vi "Project.vi"() -> ()   [LabVIEW 2015]
uses:
  <vilib>/express/express analysis/Spectral/Block/exnSpectralBlock spectral measurements RMS poly.vi
  <vilib>/express/express analysis/Spectral/Block/exnSpectralBlock spectral measurements RMS WFM.vi
  <vilib>/Analysis/BLAS.llb/dasum - Absolute Values Sum (DBL).vi
  <vilib>/express/express analysis/Spectral/XNode/ExpressSpectralMeasurementsBlockNode.xnode
  <vilib>/Analysis/NI_AALBLAS.lvlib
panel:
  out "Fourier Spectrum":cluster{"f0":dbl, "df":dbl, "magnitude":dbl[]}(graph)={"f0"=0.0, "df"=1.0, "magnitude"=[0.042500606468979685, 0.5367467757567798, 0.3916687019986553, 0.298960203892999, 0.6710643612299553, 6.999534465420016, 1.1013196943424124, 0.18951549536081805, 0.4623568704519078, 0.15713994611889348, 0.20038906279151222, 0.12934410129286392, 0.2068645394551969, 0.23302748208959884, 0.22176371644713225, 0.08751545175582917, 0.13513069757467858, 0.06308830540493562, 0.39375621048035264, 0.01345553332772048, 7.1986582467475, 0.1538936478758767, 0.11526828636783537, 0.06727117464447396, 0.2733833694778588, 0.08171771490184758, 0.12959665685604613, 0.08906888825527193, 0.2742960376602098, 0.10825189397057566, 0.09709745409455775, 0.2003023769713194, 0.24422273703495245, 0.154193230936854, 0.02225848069093769, 0.029518364210050947, 0.2694030850949449, 0.2545730206460508, 0.03493546942572119, 0.09895571125122078, 0.2284739144767194, 0.15064812633383587, 0.1284930441857229, 0.14474851518272724, 0.17923036833316625, 0.19036481120281232, 0.17636492792839045, 0.12006498175113303, 0.17954194318688638, 0.2106284617581408, 0.28299962121792593, 0.23538566157052568, 0.24018555003640282, 0.21640041472758512, 0.15124757101737055, 0.41949661945335315, 0.26981879550897725, 0.3121049852500721, 0.21283121052781867, 0.1144161007007223, 0.038379238629345995, 0.175611095155444, 0.16924306029322697, 0.12385448026581655, 0.1923464059916112, 0.07057792904819817, 0.3486628706475919, 0.2009341421247829, 0.08525005488238824, 0.20977161977382267, 0.1453650823578436, 0.1431424252882681, 0.059231936392411665, 0.13436972017141216, 0.28955881004011635, 0.07573136580325543, 0.06606205335724372, 0.14558694880418183, 0.32055634954788337, 0.22718438354488651, 0.18219262461648686, 0.19819529612638756, 0.1487142960740928, 0.19435083193650474, 0.2796530641919394, 0.2047749002206927, 0.17560519890704968, 0.0749335177489569, 0.2094618322590892, 0.22651111780504582, 0.2687989213716374, 0.05369198430782306, 0.2673345751334469, 0.0820361099822341, 0.19700727228344972, 0.15885103940219794, 0.04575621708989778, 0.16624917215261403, 0.22324613578155592, 0.187351445812392, 0.17031845157274614, 0.15605156144144403, 0.04349518882546851, 0.11015896442560126, 0.12521262552660195, 0.27256222244391815, 0.16612622567752935, 0.08331982192792557, 0.13327253312710066, 0.11820011397981438, 0.05092440172217743, 0.1562181104471463, 0.06356871067912839, 0.025291781140966803, 0.07366258187712839, 0.04899484785766527, 0.17004284219712917, 0.2291448952701625, 0.11227773245596889, 0.2590399027576651, 0.37113895563038846, 0.13688425472392202, 0.15369470064917456, 0.2433138852913691, 0.11395511628774903, 0.06992463734083774, 0.1688996669469843, 0.13321695719091933, 0.2040585097628717, 0.0956128237019304, 0.35305275146832266, 0.20659909856876377, 0.18278264472675343, 0.11862092550373249, 0.21615640903711406, 0.005466938845928891, 0.04834030072898183, 0.11810515752317857, 0.2399959977159501, 0.16182492199217044, 0.19943672319512568, 0.22908092580753284, 0.08685898392059657, 0.04446378872366921, 0.23473566824555786, 0.31932320319110064, 0.14749786785182264, 0.2035514747695043, 0.24834736430057552, 0.04732214870398398, 0.084854870790222, 0.10821838246866636, 0.052916777572832766, 0.2576431187317644, 0.31967073775982635, 0.1294961841253466, 0.21302182403480585, 0.13266721319673241, 0.20161359262642792, 0.09367318438910262, 0.2753840360773996, 0.1446051407385373, 0.19308934590941068, 0.21420985210354446, 0.11206814176593971, 0.14335589014874986, 0.20554435486158706, 0.23364898350936902, 0.1250348034876926, 0.10188274954257691, 0.19711928844012502, 0.2449897378592167, 0.14415765498295102, 0.1462160193915059, 0.2323370581534915, 0.15500869972153258, 0.13448200894013093, 0.12623430420206608, 0.0814456185216614, 0.3345455636832345, 0.12227071680153749, 0.09628364646159387, 0.026003018058545983, 0.12401400609575329, 0.07215582540361093, 0.0704208712020497, 0.05200858484906939, 0.1747832765063544, 0.09319960467240128, 0.2741746403839855, 0.11642438740239149, 0.17523938390421662, 0.17707288832102613, 0.207334292456349, 0.0631547697409838, 0.2812496049564702, 0.12804894391269359, 0.0906061842503424, 0.04263236833632178, 0.1673510435636548, 0.04851839505435179, 0.1813262929599818, 0.07621149057286354, 0.1805759327975607, 0.11838762119655057, 0.12274859651432236, 0.23680639090807448, 0.14074629473840092, 0.1603172724364417, 0.3185635367956588, 0.33209869717198015, 0.19939894848470607, 0.14352916387432882, 0.018885449815040662, 0.20622477715878493, 0.14310980408504076, 0.20355570130191603, 0.03898432313943315, 0.12766037571976296, 0.14036368255290005, 0.11777461104148834, 0.22535301463980875, 0.19671599834442935, 0.12228167253705371, 0.12841817008700945, 0.020907338638923318, 0.23426241910214296, 0.0776346836526901, 0.159518700060904, 0.27275196434096566, 0.053522107067564835, 0.2758823191052759, 0.09807878066375397, 0.4361578003469896, 0.1960268699163594, 0.14399978841629726, 0.22199792417495132, 0.2478353826994213, 0.27655766869358206, 0.20823032315513126, 0.1461218892664329, 0.09241074042943347, 0.09040897390136578, 0.07710614694817038, 0.1044945249970084, 0.13075140368574145, 0.23577229050434836, 0.08109877199303966, 0.07310661003890322, 0.24823902569866732, 0.16680068797972647, 0.049686854469804004, 0.1727304393859046, 0.07943603747519858, 0.12842830169151004, 0.22265082084335885, 0.18589225090806072, 0.17235425449973285, 0.12849580456258655, 0.17641961837853196, 0.09725808003986489, 0.09218412258919863, 0.04902416967250686, 0.047109594834610385, 0.01091093897971936, 0.12185685844942323, 0.1296071418093505, 0.34144595699972985, 0.2589951211722393, 0.18636450017521866, 0.19233542811841162, 0.20729712718056878, 0.052156728871158284, 0.1525360579854861, 0.04814771061197348, 0.2337726237323051, 0.16164341609424074, 0.14732035840907654, 0.1268852766399408, 0.18970501399979636, 0.07676131260031832, 0.0819950005333896, 0.34474780745712097, 0.06674703617025501, 0.016633110683778957, 0.12960832881619871, 0.16093955085609585, 0.18754980065189242, 0.2500408046204119, 0.32694517314858557, 0.234620989429837, 0.21799594281197146, 0.3193258265330217, 0.10799787440845852, 0.17255360786802693, 0.16461388960552076, 0.2862104274501431, 0.08916628622854066, 0.2629112652148336, 0.12240304790527766, 0.3004979186430638, 0.1671244531613923, 0.31733810119292727, 0.17650180146835942, 0.1050593685749668, 0.22793714180441585, 0.15995547357602397, 0.13332351166699732, 0.11846400545483374, 0.05000385462076186, 0.1726788788236701, 0.08940315689239495, 0.17872874860390928, 0.13578628472728713, 0.14995997188024648, 0.24466760589002684, 0.20277213852081946, 0.19574220169502107, 0.2189529456950287, 0.14660943292842446, 0.2127272107553525, 0.26947048315246674, 0.08512027917511349, 0.1211433923107559, 0.1004689906083817, 0.22881819802029907, 0.016950825622060347, 0.18029059366177966, 0.17528968961917218, 0.13622143102517612, 0.11715386128059042, 0.01761331885913314, 0.23244228221537416, 0.1882318656377289, 0.031703823228856017, 0.40954654152260783, 0.14295307169851734, 0.18076586292668276, 0.2775386000815448, 0.024134317382325875, 0.0797548675345617, 0.2150065912130813, 0.28088864194539126, 0.28869118041670677, 0.06268848695910141, 0.19553486366205974, 0.22913727951092996, 0.1469799548587168, 0.11782976288105372, 0.13123047378237396, 0.04464040970696458, 0.3056160817093, 0.09222944322592795, 0.07995288116934744, 0.13595750107057997, 0.08154619949402708, 0.2647310773940306, 0.20730755055272126, 0.1995869607556393, 0.0889189989158518, 0.37692755947524975, 0.1507077536970488, 0.14208148313320296, 0.19023300238644908, 0.13388671149828937, 0.03854906889865488, 0.09009768388512594, 0.34648566012276777, 0.040634789500672654, 0.1923827604813422, 0.024654657719097993, 0.15279339566350253, 0.27746507516145763, 0.17099964102505988, 0.15531670144052814, 0.2889627105638255, 0.10899932829815996, 0.2264683034103879, 0.20284812034305064, 0.11996889308299687, 0.0615977190337736, 0.12200964675062799, 0.084479835938092, 0.1097493304421979, 0.17068321961571548, 0.3472922373150462, 0.23130890158176834, 0.14961524033328333, 0.15267655225398805, 0.2608768035992188, 0.13623443726326545, 0.08005621863914979, 0.04637170666159416, 0.259714437725465, 0.13546363463859565, 0.29532092141764693, 0.24160138035048181, 0.2838050736564832, 0.12513176797218042, 0.10320003875502054, 0.077055460575105, 0.15177784659744586, 0.15061527206722372, 0.3056204223572756, 0.08270682277042478, 0.15458227513428863, 0.18105600456514928, 0.13806836477272233, 0.1495426690734692, 0.08660276157328292, 0.03194538924846089, 0.11970628398633147, 0.061733132929528804, 0.11722554488899106, 0.2309734783220964, 0.11207876671754691, 0.1346181820282278, 0.2980022754307246, 0.25059248357888947, 0.17727093414519776, 0.2344706806853595, 0.09206719408070126, 0.05417646298190689, 0.32763577165565594, 0.2503353797735181, 0.11241627652424947, 0.2502348756496975, 0.03769295501977679, 0.1620673513528995, 0.12362009101637524, 0.08443663244056093, 0.27766101731923254, 0.0491974260744356, 0.2561310443830817, 0.09656994710823376, 0.028176172259181623, 0.14107583573005222, 0.03448373047398869, 0.1829318430108421, 0.30285622564708364, 0.19893936900668135, 0.2950113130092603, 0.19578529440234396, 0.39470533536281244, 0.08349841817903632, 0.1416268192580781, 0.058001320791533334, 0.26806916857703195, 0.16945710851131404, 0.08921751604962813, 0.346462383750539, 0.2356040465646151, 0.16669980618123148, 0.09719474147266707, 0.027430457227979228, 0.07276273457254388, 0.08028028128394851, 0.163148873125693, 0.10062819322438275, 0.18124877934391875, 0.12555079457923954, 0.1420453479766035, 0.03595961840435948, 0.05721658653874634, 0.33170751196987674, 0.14167678950146512, 0.24694748748114168, 0.12246096447210965, 0.21744296751774353, 0.05382856500502381, 0.10105211855873389, 0.21762102654375703, 0.2789008119960079, 0.18343622651752467, 0.15300653752411209, 0.22304875012238617, 0.07901686331810699, 0.09711503371240678, 0.1462239220803364, 0.13623632806099223, 0.20720687224004106, 0.2408865465647622, 0.06442222217925131, 0.22295460236227704, 0.3840106178140434, 0.19827442315358199, 0.22593890115181264, 0.1831168361615332, 0.2805203491034643, 0.34156601639641515, 0.11414210927056462, 0.143686437840013, 0.08248917549381536, 0.2057435792845121, 0.21302248359748455, 0.1450103189960418, 0.2552407536058123, 0.2673733382279406, 0.04519425490905238, 0.20337112828894363]}
  in  "stop":bool
  out "1":bool
  out "2":bool
  out "3":bool
  out "4":bool
  out "5":bool
  out "6":bool
  out "7":bool
  out "8":bool
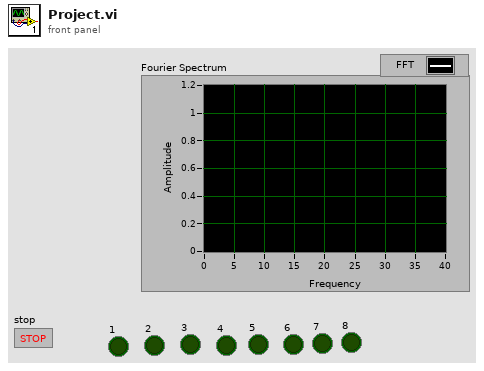
[diagram p1: front panel]
types:
  T1 = cluster{"averaging mode":u16, "weighting mode":u16, "number of averages":u32}
  T2 = cluster{"dB On (F)":bool, "unwrap phase (F)":bool, "convert to degree (F)":bool}
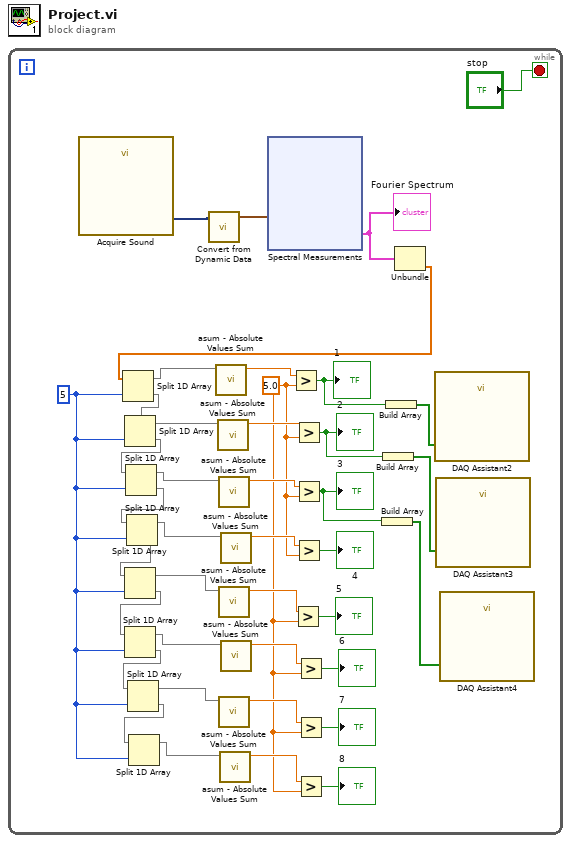
[diagram p0: block diagram]
diagram:
  n1 = while {
    stop <- "stop" stop-if-true
    w10 = 5
    w9 = 5.0 ("y")
    n2 = call "Acquire Sound"() -> ("Data"=w1:dynamicdata)  [unwired: 18 in, 1 out]
    n3 = call "Convert from Dynamic Data"("Dynamic Data Type"=w1) -> ("Waveform"=w8:waveform(dbl))  [unwired: 3 in]
    n4 = xnode "Spectral Measurements"("Signals"=w8) -> ("FFT - (RMS)"=w40:cluster{"f0":dbl, "df":dbl, "magnitude":dbl[]})  [unwired: 1 in, 2 out]
    "Fourier Spectrum" <- w40
    n5 = Unbundle(w40) -> ("magnitude"=w39:dbl[])  [unwired: 2 out]
    n6 = Split 1D Array(array=w39, index=w10) -> (first subarray=w35:dbl[], second subarray=w38:dbl[])
    n7 = Split 1D Array(array=w38, index=w10) -> (first subarray=w34:dbl[], second subarray=w37:dbl[])
    n8 = Split 1D Array(array=w37, index=w10) -> (first subarray=w33:dbl[], second subarray=w36:dbl[])
    n9 = Split 1D Array(array=w36, index=w10) -> (first subarray=w32:dbl[], second subarray=w16:dbl[])
    n10 = Split 1D Array(array=w16, index=w10) -> (first subarray=w14:dbl[], second subarray=w26:dbl[])
    n11 = Split 1D Array(array=w26, index=w10) -> (first subarray=w13:dbl[], second subarray=w25:dbl[])
    n12 = Split 1D Array(array=w25, index=w10) -> (first subarray=w23:dbl[], second subarray=w24:dbl[])
    n13 = Split 1D Array(array=w24, index=w10) -> (first subarray=w22:dbl[])  [unwired: 1 out]
    n14 = call-poly <vilib>:"asum - Absolute Values Sum.vi"("x"=w35) -> ("dasum"=w31:dbl)  [unwired: 9 in, 1 out]
    n15 = call-poly <vilib>:"asum - Absolute Values Sum.vi"("x"=w34) -> ("dasum"=w30:dbl)  [unwired: 9 in, 1 out]
    n16 = call-poly <vilib>:"asum - Absolute Values Sum.vi"("x"=w33) -> ("dasum"=w29:dbl)  [unwired: 9 in, 1 out]
    n17 = call-poly <vilib>:"asum - Absolute Values Sum.vi"("x"=w14) -> ("dasum"=w12:dbl)  [unwired: 9 in, 1 out]
    n18 = call-poly <vilib>:"asum - Absolute Values Sum.vi"("x"=w23) -> ("dasum"=w21:dbl)  [unwired: 9 in, 1 out]
    n19 = call-poly <vilib>:"asum - Absolute Values Sum.vi"("x"=w22) -> ("dasum"=w20:dbl)  [unwired: 9 in, 1 out]
    n20 = call-poly <vilib>:"asum - Absolute Values Sum.vi"("x"=w32) -> ("dasum"=w28:dbl)  [unwired: 9 in, 1 out]
    n21 = call-poly <vilib>:"asum - Absolute Values Sum.vi"("x"=w13) -> ("dasum"=w11:dbl)  [unwired: 9 in, 1 out]
    n22 = Greater?(x=w31, y=w9) -> (0:w7:bool)
    "1" <- w7
    n23 = Greater?(x=w12, y=w9) -> (0:→"5":bool)
    n24 = Greater?(x=w30, y=w9) -> (0:w5:bool)
    "2" <- w5
    n25 = Greater?(x=w29, y=w9) -> (0:w3:bool)
    "3" <- w3
    n26 = Greater?(x=w28, y=w9) -> (0:→"4":bool)
    n27 = Greater?(x=w11, y=w9) -> (0:→"6":bool)
    n28 = Greater?(x=w21, y=w9) -> (0:→"7":bool)
    n29 = Greater?(x=w20, y=w9) -> (0:→"8":bool)
    n30 = Build Array(w3) -> (w2:bool[])
    n31 = Build Array(w5) -> (w4:bool[])
    n32 = Build Array(w7) -> (w6:bool[])
    n33 = call "DAQ Assistant2"("data"=w6) -> ()  [unwired: 17 in, 2 out]
    n34 = call "DAQ Assistant3"("data"=w4) -> ()  [unwired: 17 in, 2 out]
    n35 = call "DAQ Assistant4"("data"=w2) -> ()  [unwired: 17 in, 2 out]
  }
